vi "czujka.vi"(7 "LabVIEW Web Service Request":refnum<class "Web Request.lvclass">, 11 "waveform in":waveform(dbl)) -> (2 "dane poprawione":string, 3 "dane":string)   [LabVIEW 2018]
uses:
  <vilib>/wsapi/Web Request.lvclass
panel:
  out "data":string
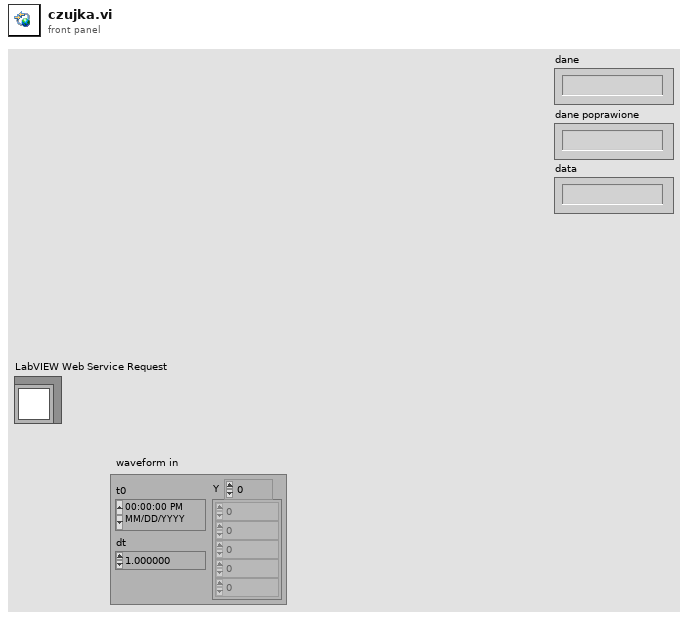
[diagram p1: front panel]
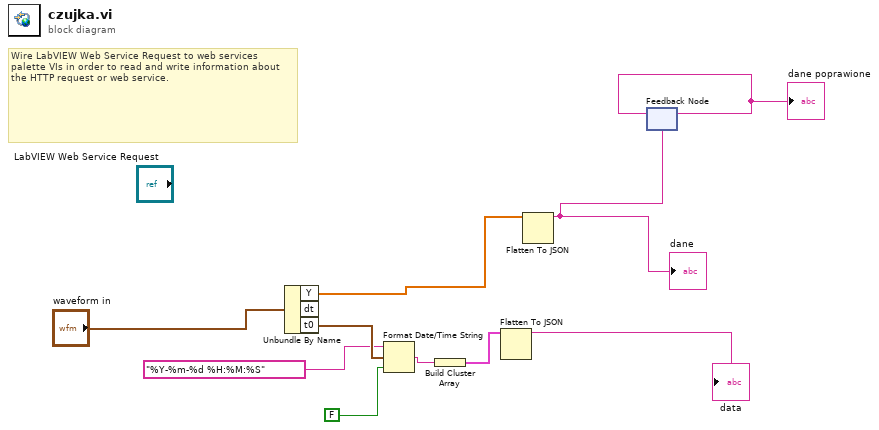
[diagram p0: block diagram]
diagram:
  # "Wire LabVIEW Web Service Request to web services palette VIs in order to read and write information about the HTTP request or web service."
  n1 = Unbundle By Name("waveform in") -> ("Y"=w7:dbl[], "t0"=w9:timestamp)  [unwired: 1 out]
  n2 = Format Date/Time String(time format string (%c)="%Y-%m-%d %H:%M:%S", seconds (now)=w9, UTC format=FALSE) -> (date/time string=w5:string)
  n3 = Build Cluster Array(w5) -> (w4:cluster{"date/time string":string}[])
  n4 = Flatten To JSON(anything=w4) -> (JSON string=→"data":string)  [unwired: 2 in, 1 out]
  n5 = Flatten To JSON(anything=w7) -> (JSON string=w1:string)  [unwired: 2 in, 1 out]
  "dane" <- w1
  n6 = feedback #1(w1) -> (w2:string)
  "dane poprawione" <- w2
  n7 = feedback-in #1(w2) -> ()
